vi "streaming_x502.vi"() -> ()   [LabVIEW 2012]
panel:
  in  "SyncMode":u32(ring) items=["INTERNAL"=0, "EXTERNAL_MASTER"=1, "DI_SYN1_RISE"=2, "DI_SYN1_FALL"=3, "DI_SYN2_RISE"=6, "DI_SYN2_FALL"=7]
  out "error out":errorcluster
  in  "error in (no error)":errorcluster
  in  "Offset_I":dbl
  in  "Coeff_I":dbl=42.391
  out "din_data_size":u32
  in  "Offset_U":dbl
  in  "Coeff_U":dbl=2.55
  out "Time_indicator":dbl format="%.1f"
  out "Ток":dbl[](graph)
  out "Напряжение":dbl[](graph)
  in  "Стоп":bool
  out "DIN":u32[](array[numeric]) format="%b"
  in  "IP Addr":string="192.168.0.1"
  out "MCU ver":string
  in  "Отображать за время":dbl=100.0 min=10.0 step=1.0
  out "Установленная частота синхронного ввода DIN":dbl=2.0 min=2.0 max=2000000.0 format="%#_8f"
  in  "Частота синхронного ввода DIN":dbl=20000.0 min=1.0 max=2000000.0 format="%#_8f"
  out "FPGA Ver":string
  out "Установленная частота на канал":dbl=2.0 min=2.0 max=2000000.0 format="%#_8f"
  out "Установленная частота сбора":dbl=2.0 min=2.0 max=2000000.0 format="%#_8f"
  in  "Частота сбора на канал":dbl=50000.0 min=2.0 max=2000000.0 format="%#_8f"
  in  "Частота сбора (Гц)":dbl=100000.0 min=2.0 max=2000000.0 format="%#_8f"
  out "PldaVer":u8
  out "Serial":string
  out "Name":string
  # "Информация о плате"
  # "Настройки модуля"
  # "Устанавливаемое"
  # "Установленное"
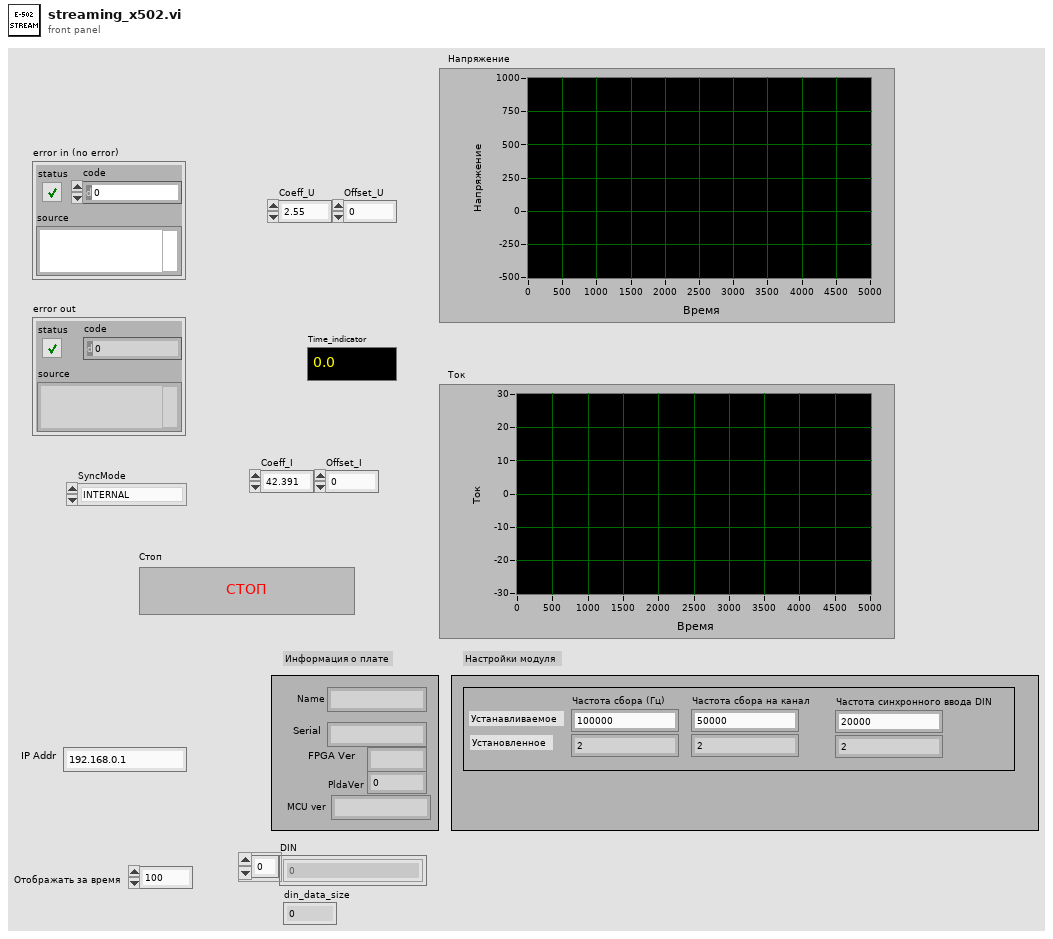
[diagram p1: front panel]
types:
  T1 = cluster{"PhyCh":u32, "Avg":u32, "Mode":u32, "Range":u32}[]
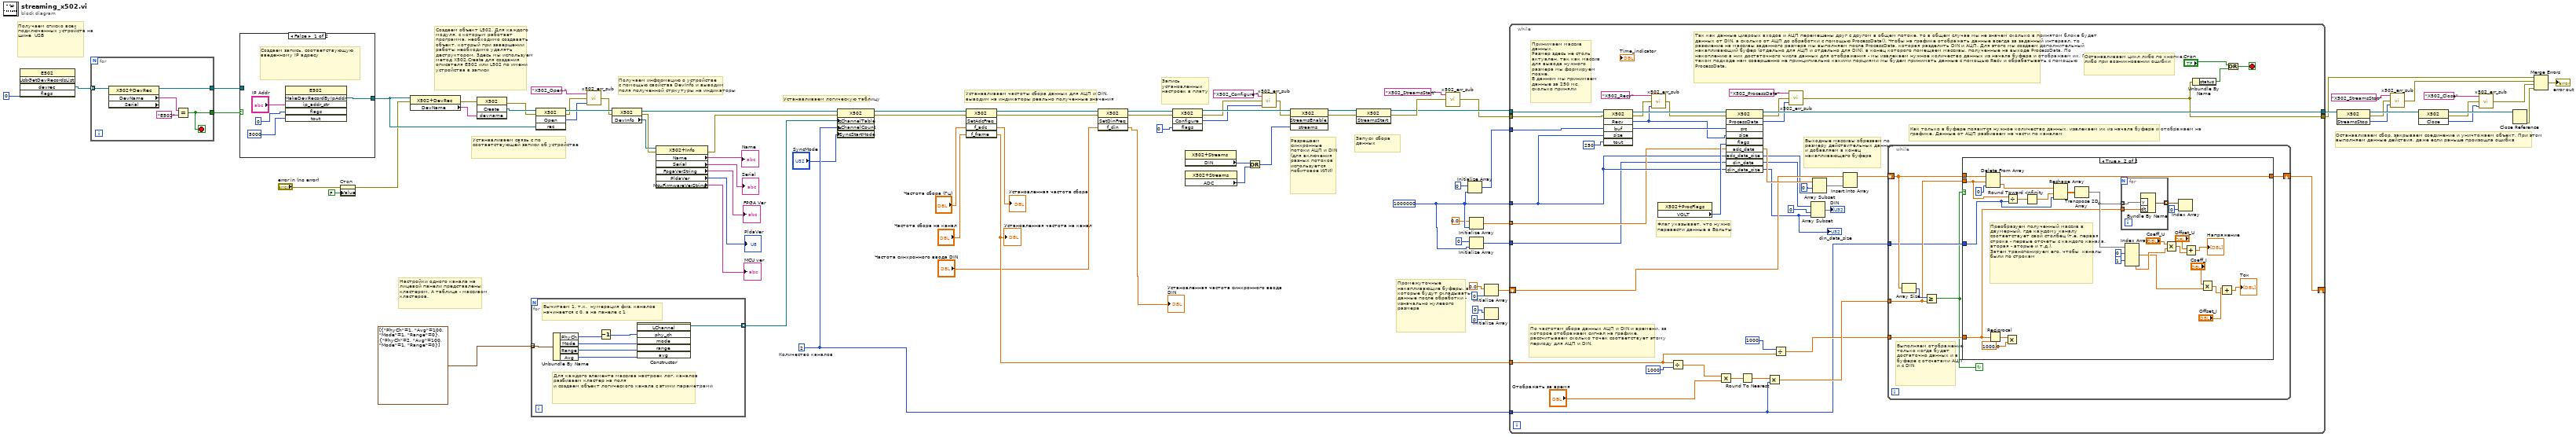
[diagram p0: block diagram]
diagram:
  w83 = u32 2  # Количество каналов
  w78 = u32 1000000 ("element")
  # "Получаем списко всех подключенных устройств на шине  USB"
  # "Останавливаем сбор, закрываем соединение и уничтожаем объект. При этом выполняем данные действия, даже если раньше произошла ошибка"
  # "Промежуточные накапливающие буферы, в которые будут складываться данные после обработки - изначально нулевого размера"
  # "Запуск сбора данных"
  # "Разрешаем синхронные потоки АЦП и DIN (для включения разных потоков используется побитовое ИЛИ)"
  # "Запись установленных настроек в плату"
  # "Устанавливаем частоты сбора данных для АЦП и DIN,\nвыводим на индикаторы реально полученные значения"
  # "Устанавливаем логическую таблицу"
  # "Настройки одного канала на лицевой панели представлены кластером. А таблица - массивом кластеров."
  # "Создаем объект L502. Для каждого модуля, с которым работает программа, необходимо создавать объект, который при завершении работы необходимо удалять деструктором. Здесь мы используем метод X502.Create для создания описателя E502 или L502 по имени устройства в записи"
  # "Получаем информацию о устройстве \nс помощью свойства DevInfo и выводим\nполя полученной стркутуры на индикаторы"
  # "Устанавливаем связь с по соответствующей записи об устройстве"
  n1 = invoke class="E502" method="UsbGetDevRecordsList"("flags"=0) -> ("devrec"=w6:refnum<k24>[])  [unwired: 4 in, 4 out]
  n2 = for {
    tunnel: w6 -> [w88] mode=indexing
    tunnel: [w87] -> w4
    tunnel: [w84] -> w5
    stop <- w84 stop-if-true
    n3 = property class="X502+DevRec" props=["DevName", "Serial"](reference=w88) -> (reference out=w87:refnum<k24>, "DevName"=w86:string)  [unwired: 1 in, 2 out]
    n4 = Equal?(x=w86, y="E502") -> (x = y?=w84:bool)
  }
  n5 = case shown="False" w5 {
    tunnel: [w89 w93] -> w15
    tunnel: w4 -> [_ w93]
    frame False {
      # "Создаем запись, соответствующую введенному IP адресу"
      n6 = invoke class="E502" method="MakeDevRecordByIpAddr"("ip_addr_str"="IP Addr", "flags"=0, "tout"=5000) -> ("MakeDevRecordByIpAddr"=w89:refnum<k24>)  [unwired: 3 in, 5 out]
    }
    frame True {
    }
  }
  n7 = property on="Стоп" class="Bool (strict)"(error in="error in (no error)", "Value"=FALSE ("Стоп")) -> (error out=w8:errorcluster)  [unwired: 1 in, 1 out]
  n8 = property class="X502+DevRec"(reference=w15, error in=w8) -> (error out=w10:errorcluster, "DevName"=w46:string)  [unwired: 1 out]
  n9 = invoke class="X502" method="Create"(error in=w10, "devname"=w46) -> (error out=w45:errorcluster, "Create"=w47:refnum<k24>)  [unwired: 2 in, 2 out]
  n10 = for {
    tunnel: T1 [{"PhyCh"=1, "Avg"=100, "Mode"=1, "Range"=0}, {"PhyCh"=2, "Avg"=100, "Mode"=1, "Range"=0}] ("Логические каналы") -> [w100] mode=indexing
    tunnel: [w94] -> w72 mode=indexing
    # "Вычитаем 1, т.к.  нумерация физ. каналов начинается с 0, а на панеле с 1"
    # "Для каждого элемента массива настроек лог. каналов разбиваем кластер на поля\nи создаем объект логического канала с этими параметрами"
    n11 = Unbundle By Name(w100) -> ("PhyCh"=w99:u32, "Mode"=w97:u32, "Range"=w96:u32, "Avg"=w95:u32)
    n12 = Decrement(x=w99) -> (x-1=w98:u32)
    n13 = constructor class="X502+LChannel"("phy_ch"=w98, "mode"=w97, "range"=w96, "avg"=w95) -> (reference out=w94:refnum<k24>)  [unwired: 3 in, 6 out]
  }
  n14 = invoke class="X502" method="Open"(reference=w47, error in=w45, "rec"=w15) -> (reference out=w50:refnum<k24>, error out=w43:errorcluster, "Open"=w44:i32)  [unwired: 1 in, 1 out]
  n15 = call "x502_err_sub.vi"("Error code"=w44, "error in (no error)"=w43, "Error descr"="X502_Open ") -> ("error out"=w41:errorcluster)
  n16 = property class="X502"(reference=w50, error in=w41) -> (reference out=w51:refnum<k24>, error out=w39:errorcluster, "DevInfo"=w40:refnum<k24>)
  n17 = property class="X502+Info"(reference=w40, error in=w39) -> (error out=w16:errorcluster, "Name"=→"Name":string, "Serial"=→"Serial":string, "FpgaVerString"=→"FPGA Ver":string, "PldaVer"=→"PldaVer":u8, "McuFirmwareVerString"=→"MCU ver":string)  [unwired: 1 out]
  n18 = property class="X502"(reference=w51, error in=w16, "LChannelTable"=w72, "LChannelCount"=w83, "SyncStartMode"="SyncMode") -> (reference out=w52:refnum<k24>, error out=w53:errorcluster)
  n19 = invoke class="X502" method="SetAdcFreq"(reference=w52, error in=w53, "f_adc"="Частота сбора (Гц)", "f_frame"="Частота сбора на канал") -> (reference out=w57:refnum<k24>, error out=w58:errorcluster, "f_adc"=→"Установленная частота сбора":dbl, "f_frame"=w75:dbl)  [unwired: 1 in, 1 out]
  "Установленная частота на канал" <- w75
  n20 = invoke class="X502" method="SetDinFreq"(reference=w57, error in=w58, "f_din"="Частота синхронного ввода DIN") -> (reference out=w62:refnum<k24>, error out=w63:errorcluster, "f_din"=→"Установленная частота синхронного ввода DIN":dbl)  [unwired: 1 in, 1 out]
  n21 = invoke class="X502" method="Configure"(reference=w62, error in=w63, "flags"=0) -> (reference out=w64:refnum<k24>, error out=w33:errorcluster, "Configure"=w31:i32)  [unwired: 1 in, 1 out]
  n22 = property class="X502+Streams"() -> ("DIN"=w25:u32)  [unwired: 2 in, 2 out]
  n23 = property class="X502+Streams"() -> ("ADC"=w61:u32)  [unwired: 2 in, 2 out]
  n24 = Or(x=w25, y=w61) -> (x .or. y?=w24:u32)
  n25 = call "x502_err_sub.vi"("Error code"=w31, "error in (no error)"=w33, "Error descr"="X502_Configure ") -> ("error out"=w32:errorcluster)
  n26 = invoke class="X502" method="StreamsEnable"(reference=w64, error in=w32, "streams"=w24) -> (reference out=w65:refnum<k24>, error out=w66:errorcluster)  [unwired: 1 in, 2 out]
  n27 = invoke class="X502" method="StreamsStart"(reference=w65, error in=w66) -> (reference out=w27:refnum<k24>, error out=w29:errorcluster)  [unwired: 1 in, 1 out]
  n28 = call "x502_err_sub.vi"("error in (no error)"=w29, "Error descr"="X502_StreamsStart") -> ("error out"=w26:errorcluster)  [unwired: 1 in]
  n29 = Initialize Array(u32 0 ("element"), w78) -> (w79:u32[])
  n30 = Initialize Array(0.0 ("element"), w78) -> (w81:dbl[])
  n31 = Initialize Array(u32 0 ("element"), w78) -> (w80:u32[])
  n32 = Initialize Array(0.0 ("element"), u32 0 ("element")) -> (w82:dbl[])
  n33 = Initialize Array(u32 0 ("element"), u32 0 ("element")) -> ()  [unwired: 1 out]
  n34 = while {
    tunnel: w27 -> [w143]
    tunnel: w26 -> [w142]
    tunnel: [w141] -> w23
    tunnel: w79 -> [w140]
    shift-right: [w135] -> _
    shift-left: w82 -> [w134]
    tunnel: w83 -> [w104]
    tunnel: w75 -> [w117]
    tunnel: w78 -> [w116]
    tunnel: w80 -> [w102]
    tunnel: w81 -> [w115]
    tunnel: [w105] -> w11
    stop <- w119 stop-if-true
    # "Так как данные цивроых входов и АЦП перемешены друг с другом в общем потоке, то в общем случае мы не значем сколько в принятом блоке будет данных от DIN, а сколько от АЦП до обработки с помощью ProcessData(). Чтобы на графике отображать данные всегда за заданный интервал, то разюиение на массивы заданного размера мы выполняем после ProcessData, которая разделить DIN и АЦП. Для этого мы создаем дополнительный накапливающий буфер (отдельно для АЦП и отдельно для DIN), в конец которого помещаем массивы, полученные на выходе ProcessData. По накоплению в них достаточного числа данных для отображения - мы извлекаем нужное количество данных из начала буфера и отображаем их. При таком подходе нам совершенно не принципиально какими порциями мы будем принимать данные с помощью Recv и обрабатывать с помощью ProcessData."
    # "Останавливаем цикл либо по кнопке, либо при возникновении ошибки"
    # "Как только в буфере появится нужное количество данных, извлекаем их из начала буфера и отображаем на графике. Данные от АЦП разбиваем на части по каналам"
    # "По частотам сбора данных АЦП и DIN и времени, за которое отображаем сигнал на графике, рассчитываем сколько точек соответствует этому периоду для АЦП и DIN."
    # "Выходные массивы обрезаем по размеру действительных данных и добавляем в конец накапливающего буфера"
    # "Флаг указывает, что нужно перевести данные в Вольты"
    # "Принимаем массив данных.\nРазмер здесь не столь актуален, так как массив для вывода нужного размера мы формируем позже.\nВ данном мы принимаем данные за 250 мс, сколько приняли"
    n35 = invoke class="X502" method="Recv"(reference=w143, error in=w142, "buf"=w140, "size"=w116, "tout"=u32 250 ("element")) -> (reference out=w131:refnum<k24>, error out=w112:errorcluster, "Recv"=w111:i32, "buf"=w139:u32[])  [unwired: 1 in, 2 out]
    n36 = call "x502_err_sub.vi"("Error code"=w111, "error in (no error)"=w112, "Error descr"="X502_Recv") -> ("error out"=w110:errorcluster)
    n37 = property class="X502+ProcFlags"() -> ("VOLT"=w130:u32)  [unwired: 2 in, 2 out]
    n38 = Divide(x=w117, y=1000) -> (x/y=w124:dbl)
    n39 = Multiply(x=w124, y="Отображать за время") -> (x*y=w123:dbl)
    n40 = invoke class="X502" method="ProcessData"(reference=w131, error in=w110, "src"=w139, "size"=w111, "flags"=w130, "adc_data"=w115, "adc_data_size"=w116, "din_data"=w102, "din_data_size"=w116) -> (reference out=w141:refnum<k24>, error out=w108:errorcluster, "ProcessData"=w107:i32, "adc_data"=w137:dbl[], "adc_data_size"=w132:u32, "din_data"=w127:u32[], "din_data_size"=w126:u32)  [unwired: 1 in, 3 out]
    "din_data_size" <- w126
    n41 = Round To Nearest(number=w123) -> (nearest integer value=w122:dbl)
    n42 = Multiply(x=w122, y=w104) -> (x*y=w120:dbl)
    n43 = Divide(x=u32 1000 ("element"), y=w117) -> (x/y=w114:dbl)
    n44 = call "x502_err_sub.vi"("Error code"=w107, "error in (no error)"=w108, "Error descr"="X502_ProcessData") -> ("error out"=w105:errorcluster)
    n45 = Array Subset(array=w127, index=u32 0 ("element"), length=w126) -> (→"DIN":u32[])
    n46 = Array Subset(array=w137, index=u32 0 ("element"), length=w132) -> (w129:dbl[])
    n47 = Insert Into Array(array=w134, new element=w129) -> (w133:dbl[])  [unwired: 1 in]
    n48 = while {
      shift-right: [w150] -> w135
      shift-left: w133 -> [w149]
      tunnel: w120 -> [w147]
      tunnel: w114 -> [w146]
      tunnel: w104 -> [w145]
      stop <- w144 continue-if-true
      # "Выполняем отображение только когда будет достаточно данных и в буфере с отсчетами АЦП и с DIN"
      n49 = Array Size(array=w149) -> (size(s)=w148:i32)
      n50 = Greater Or Equal?(x=w148, y=w147) -> (x >= y?=w144:bool)
      n51 = case shown="True" w144 {
        tunnel: [w151 w178] -> w150
        tunnel: w149 -> [w151 w177]
        tunnel: w147 -> [_ w173]
        tunnel: w146 -> [_ w154]
        tunnel: w145 -> [_ w171]
        frame False {
        }
        frame True {
          # "Преобразуем полученный массив в двумерный, где каждому каналу соответствует свой столбец (т.е. первая строка - первые отсчеты с каждого канала, вторая - вторые и т.д.).\nЗатем транспонируем его, чтобы  каналы были по строкам"
          n52 = Delete From Array(array=w177, length=w173, index=u32 0 ("element")) -> (deleted portion=w172:dbl[], array with subset deleted=w178:dbl[])
          n53 = Reciprocal(x=w154) -> (1/x=w153:dbl)
          n54 = Multiply(x=w153, y=1000.0) -> ()  [unwired: 1 out]
          n55 = Divide(x=w173, y=w171) -> (x/y=w175:dbl)
          n56 = Round Toward -Infinity(1:w175) -> (0:w174:dbl)
          n57 = Reshape Array(w172, w174, w171) -> (w160:dbl[][])
          n58 = Transpose 2D Array(2D array=w160) -> (transposed array=w159:dbl[][])
          n59 = for {
            tunnel: w159 -> [w180] mode=indexing
            tunnel: w154 -> [w181]
            tunnel: [w179] -> w157 mode=indexing
            n60 = Bundle By Name("Y"=w180, "dt"=w181) -> (w179:waveform(dbl))  [unwired: 1 in]
          }
          n61 = Index Array(array=w159, index (row) #1=0 ("index (row)"), index (row) #2=1 ("index (row)")) -> (element #1=w155:dbl[], element #2=w158:dbl[])  [unwired: 2 in]
          n62 = Multiply(x="Coeff_U", y=w158) -> (x*y=w164:dbl[])
          n63 = Index Array(array=w157, index=0) -> ()  [unwired: 1 out]
          n64 = Add(x="Offset_U", y=w164) -> (x+y=→"Напряжение":dbl[])
          n65 = Multiply(x="Coeff_I", y=w155) -> (x*y=w165:dbl[])
          n66 = Add(x="Offset_I", y=w165) -> (x+y=→"Ток":dbl[])
        }
      }
    }
    n67 = Unbundle By Name(w105) -> ("status"=w106:bool)
    n68 = Or(x="Стоп", y=w106) -> (x .or. y?=w119:bool)
  }
  n69 = invoke class="X502" method="StreamsStop"(reference=w23) -> (reference out=w48:refnum<k24>, error out=w22:errorcluster, "StreamsStop"=w20:i32)  [unwired: 2 in]
  n70 = call "x502_err_sub.vi"("Error code"=w20, "error in (no error)"=w22, "Error descr"="X502_StreamsStop") -> ("error out"=w12:errorcluster)
  n71 = invoke class="X502" method="Close"(reference=w48) -> (reference out=w49:refnum<k24>, error out=w18:errorcluster, "Close"=w17:i32)  [unwired: 2 in]
  n72 = call "x502_err_sub.vi"("Error code"=w17, "error in (no error)"=w18, "Error descr"="X502_Close") -> ("error out"=w13:errorcluster)
  n73 = Close Reference(reference=w49) -> (error out=w14:errorcluster)  [unwired: 1 in]
  n74 = Merge Errors(w11, w12, w13, w14) -> (→"error out":errorcluster)
